vi "FFT_curve_fit.vi"(8 "# of Fourrier coefficents":i32, 9 "# samples":i32, 10 "dt":dbl, 11 "Signal":dbl[](array[numeric])) -> ()   [LabVIEW 2012]
uses:
  <vilib>/gmath/NumericalOptimization/stopping criteria.ctl
  Controls/FFT_curve_fit_TD.ctl
  <vilib>/Utility/error.llb/DialogType.ctl
  <vilib>/Analysis/1siggen.llb/Ramp Pattern by Samples.vi
  <vilib>/gmath/NumericalOptimization/Downhill Simplex.vi
  <vilib>/Analysis/NI_AALPro.lvlib
  <vilib>/gmath/NI_Gmath.lvlib
  <vilib>/Analysis/NI_AALBase.lvlib
panel:
  out "XY Graph 3":cluster{"Ramp Pattern":dbl[], "X":dbl[]}[](graph)
  out "XY Graph 2":cluster{"Ramp Pattern":dbl[], "X":dbl[]}[](graph)
  out "XY Graph":cluster{"Ramp Pattern":dbl[], "X":dbl[]}[](graph)
  out "f(minimum)":dbl
  in  "stopping criteria":T1={"function tolerance"=1e-06, "parameter tolerance"=1e-06, "max iterations"=100, "max function calls"=1000, "gradient tolerance"=1e-06, "max time (sec)"=-1.0}
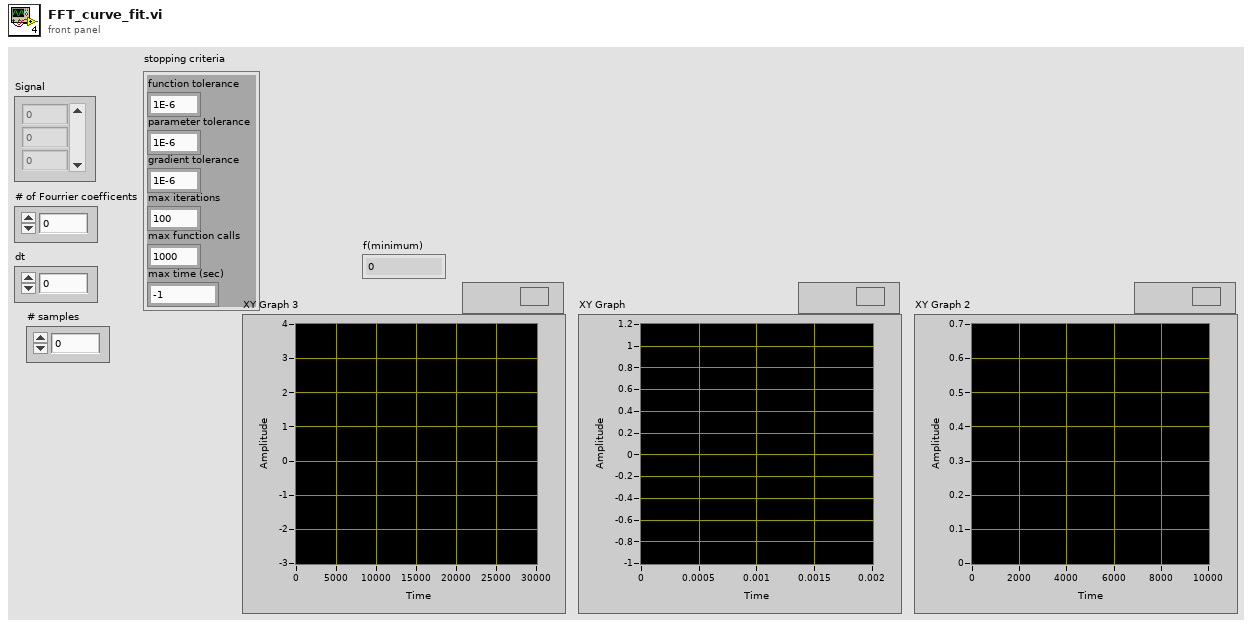
[diagram p1: front panel]
types:
  T1 = typedef "NI_Gmath.lvlib/stopping criteria.ctl" = cluster{"function tolerance":dbl, "parameter tolerance":dbl, "max iterations":i32, "max function calls":i32, "gradient tolerance":dbl, "max time (sec)":dbl}
  T2 = typedef "DialogType.ctl" = u16
  T3 = typedef "FFT_curve_fit_TD.ctl" = cluster{"Signal":dbl[], "Frequencies":dbl[], "ti":dbl[], "t":dbl[]}
  T4 = cluster{"Ramp Pattern":dbl[], "Amp Spectrum Phase (radians)":dbl[]}
  T5 = cluster{"Ramp Pattern":dbl[], "Amp Spectrum Mag (Vrms)":dbl[]}
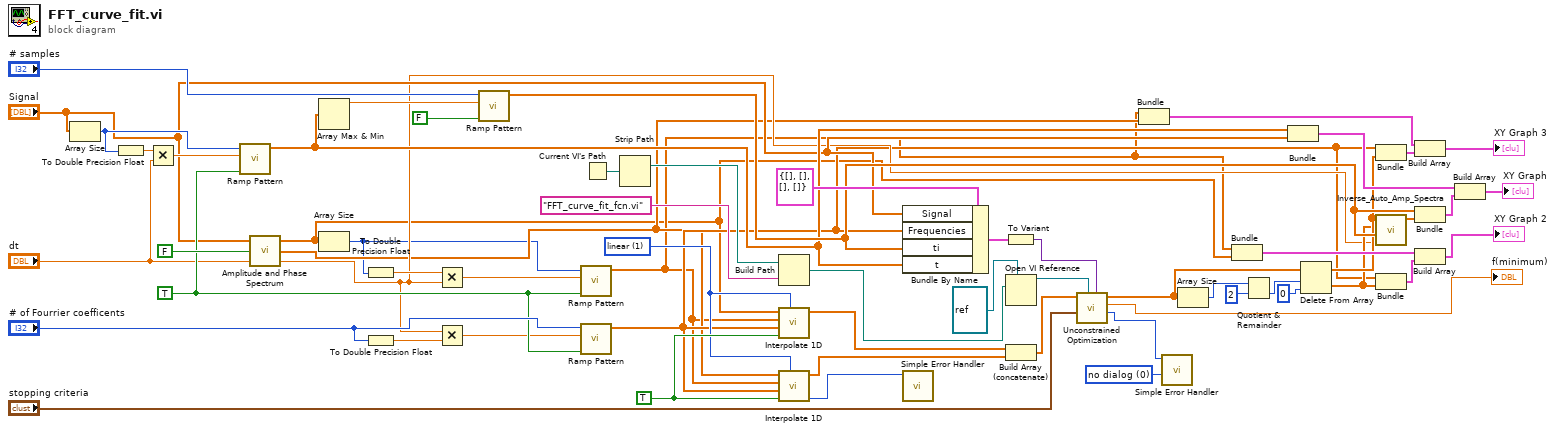
[diagram p0: block diagram]
diagram:
  w1 = T2 0 items=["no dialog", "OK message", "continue or stop message", "OK message + warnings", "continue/stop + warnings"] ("type of dialog (OK msg:1)")
  w12 = 1 items=["nearest", "linear", "spline", "cubic Hermite", "Lagrange"] ("method")
  w13 = TRUE ("X is monotonic")
  w42 = TRUE ("exclude end?")
  n1 = Array Size(array="Signal") -> (size(s)=w40:i32)
  n2 = To Double Precision Float(number=w40) -> (double precision float=w44:dbl)
  n3 = Multiply(x=w44, y="dt") -> (x*y=w38:dbl)
  n4 = call-poly <vilib>:"Ramp Pattern.vi"("exclude end?"=w42, "end"=w38, "samples"=w40) -> ("Ramp Pattern"=w27:dbl[])  [unwired: 7 in, 1 out]
  n5 = call <vilib>:"Amplitude and Phase Spectrum.vi"("dt"="dt", "unwrap phase (T)"=FALSE, "Signal (V)"="Signal") -> ("df"=w14:dbl, "Amp Spectrum Phase (radians)"=w10:dbl[], "Amp Spectrum Mag (Vrms)"=w5:dbl[])
  n6 = Array Max & Min(array=w27) -> (max value=w37:dbl)  [unwired: 3 out]
  n7 = Array Size(array=w5) -> (size(s)=w3:i32)
  n8 = To Double Precision Float(number=w3) -> (double precision float=w57:dbl)
  n9 = To Double Precision Float(number="# of Fourrier coefficents") -> (double precision float=w56:dbl)
  n10 = Multiply(x=w57, y=w14) -> (x*y=w43:dbl)
  n11 = Multiply(x=w14, y=w56) -> (x*y=w30:dbl)
  n12 = call-poly <vilib>:"Ramp Pattern.vi"("exclude end?"=FALSE, "end"=w37, "samples"="# samples") -> ("Ramp Pattern"=w28:dbl[])  [unwired: 7 in, 1 out]
  n13 = call-poly <vilib>:"Ramp Pattern.vi"("exclude end?"=w42, "end"=w43, "samples"=w3) -> ("Ramp Pattern"=w6:dbl[])  [unwired: 7 in, 1 out]
  n14 = call-poly <vilib>:"Ramp Pattern.vi"("exclude end?"=w42, "end"=w30, "samples"="# of Fourrier coefficents") -> ("Ramp Pattern"=w11:dbl[])  [unwired: 7 in, 1 out]
  n15 = Current VI's Path() -> (path=w49:path)
  n16 = Strip Path(path=w49) -> (stripped path=w48:path)  [unwired: 1 out]
  n17 = Build Path(base path=w48, name or relative path="FFT_curve_fit_fcn.vi") -> (appended path=w47:path)
  n18 = call <vilib>:"Interpolate 1D.vi"("method"=w12, "X is monotonic"=w13, "xi"=w11, "X"=w6, "Y"=w5) -> ("yi"=w9:dbl[])  [unwired: 4 in, 2 out]
  n19 = call <vilib>:"Interpolate 1D.vi"("method"=w12, "X is monotonic"=w13, "xi"=w11, "X"=w6, "Y"=w10) -> ("error"=w4:i32, "yi"=w8:dbl[])  [unwired: 4 in, 1 out]
  n20 = Bundle By Name(cluster=T3 {"Signal"=[], "Frequencies"=[], "ti"=[], "t"=[]} ("Cluster"), "Signal"="Signal", "Frequencies"=w11, "ti"=w28, "t"=w27) -> (w52:T3)
  n21 = call <vilib>:"Simple Error Handler.vi"("error code (no error:0)"=w4) -> ()  [unwired: 4 in, 5 out]
  n22 = To Variant(anything=w52) -> (Variant=w53:variant)
  n23 = Open VI Reference(type specifier VI Refnum (for type only)=refnum<vi> refnum, vi path=w47) -> (vi reference=w51:refnum<vi>)  [unwired: 4 in, 1 out]
  n24 = Build Array (concatenate)(w9, w8) -> (w7:dbl[])
  n25 = call-poly <vilib>:"Unconstrained Optimization.vi"("function data"=w53, "objective function"=w51, "stopping criteria"="stopping criteria", "start"=w7) -> ("number of function evaluations"=w2:i32, "f(minimum)"=→"f(minimum)":dbl, "minimum"=w31:dbl[])  [unwired: 4 in, 1 out]
  n26 = Bundle("Ramp Pattern"=w6, "Amp Spectrum Phase (radians)"=w10) -> (w19:T4)  [unwired: 1 in]
  n27 = call <vilib>:"Simple Error Handler.vi"("error code (no error:0)"=w2, "type of dialog (OK msg:1)"=w1) -> ()  [unwired: 3 in, 5 out]
  n28 = Array Size(array=w31) -> (size(s)=w32:i32)
  n29 = Bundle("Ramp Pattern"=w6, "Amp Spectrum Mag (Vrms)"=w5) -> (w20:T5)  [unwired: 1 in]
  n30 = Quotient & Remainder(x=w32, y=2) -> (floor(x/y)=w34:i32)  [unwired: 1 out]
  n31 = Bundle("Ramp Pattern"=w27, "Signal"="Signal") -> (w25:cluster{"Ramp Pattern":dbl[], "Signal":dbl[]})  [unwired: 1 in]
  n32 = Delete From Array(array=w31, length=w34, index=0) -> (deleted portion=w16:dbl[], array with subset deleted=w18:dbl[])
  n33 = Bundle("Ramp Pattern"=w11, "minimum"=w18) -> (w17:cluster{"Ramp Pattern":dbl[], "minimum":dbl[]})  [unwired: 1 in]
  n34 = call "Inverse_Auto_Amp_Spectra.vi"("df"=w14, "t"=w28, "Amp Spectrum Mag (Vrms)"=w16, "Amp Spectrum Phase (radians)"=w18) -> ("X"=w29:dbl[])  [unwired: 6 in, 1 out]
  n35 = Bundle("Ramp Pattern"=w11, "minimum"=w16) -> (w15:cluster{"Ramp Pattern":dbl[], "minimum":dbl[]})  [unwired: 1 in]
  n36 = Build Array(w19, w17) -> (→"XY Graph 3":cluster{"Ramp Pattern":dbl[], "minimum":dbl[]}[])
  n37 = Bundle("Ramp Pattern"=w28, "X"=w29) -> (w24:cluster{"Ramp Pattern":dbl[], "X":dbl[]})  [unwired: 1 in]
  n38 = Build Array(w20, w15) -> (→"XY Graph 2":cluster{"Ramp Pattern":dbl[], "minimum":dbl[]}[])
  n39 = Build Array(w25, w24) -> (→"XY Graph":cluster{"Ramp Pattern":dbl[], "X":dbl[]}[])
